vi "set num to enum.vi"(11 "Numeric in":u8) -> (3 "Numeric out":T1)   [LabVIEW 2021]
uses:
  mode_type.ctl
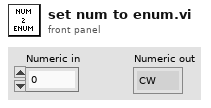
[diagram p1: front panel]
types:
  T1 = typedef "mode_type.ctl" = enum8{"CW", "NC - CW", "NC - cw", "LFM", "BPSK", "QPSK"}
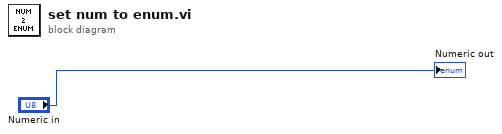
[diagram p0: block diagram]
diagram:
  "Numeric out" <- "Numeric in"
